vi "DetSim.vi"() -> ()   [LabVIEW 2011]
panel:
  out "Counting?":bool
  out "Count Value":dbl
  in  "stop program":bool
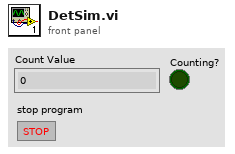
[diagram p1: front panel]
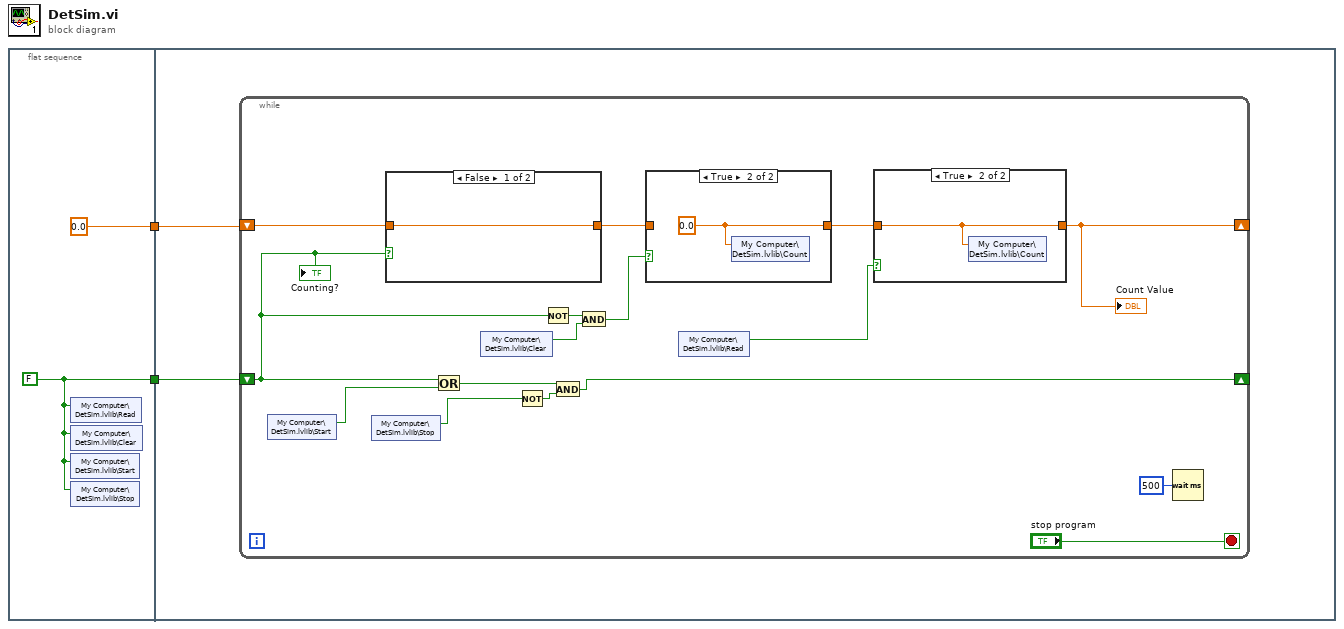
[diagram p0: block diagram]
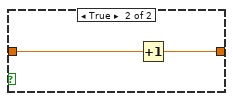
[diagram p4: hidden frame]
diagram:
  n1 = flat-sequence {
    tunnel: [0.0] -> w2
    tunnel: [w3] -> w1
    tunnel: w2 -> [w6]
    tunnel: w1 -> [w5]
    frame #0 {
      w3 = FALSE
      n2 = shared-variable "My Computer\\DetSim.lvlib\\Read"(w3) -> ()  [unwired: 1 in, 1 out]
      n3 = shared-variable "My Computer\\DetSim.lvlib\\Clear"(w3) -> ()  [unwired: 1 in, 1 out]
      n4 = shared-variable "My Computer\\DetSim.lvlib\\Start"(w3) -> ()  [unwired: 1 in, 1 out]
      n5 = shared-variable "My Computer\\DetSim.lvlib\\Stop"(w3) -> ()  [unwired: 1 in, 1 out]
    }
    frame #1 {
      n6 = while {
        shift-right: [w12] -> _
        shift-left: w6 -> [w20]
        shift-right: [w18] -> _
        shift-left: w5 -> [w14]
        stop <- "stop program" stop-if-true
        n7 = shared-variable "My Computer\\DetSim.lvlib\\Start"() -> (w10:bool)  [unwired: 1 in, 1 out]
        n8 = shared-variable "My Computer\\DetSim.lvlib\\Stop"() -> (w9:bool)  [unwired: 1 in, 1 out]
        n9 = case shown="False" w14 {
          tunnel: w20 -> [w27 w29]
          tunnel: [w27 w28] -> w16
          frame False {
          }
          frame True {
            n10 = Increment(x=w29) -> (x+1=w28:dbl)
          }
        }
        n11 = Or(x=w14, y=w10) -> (x .or. y?=w19:bool)
        n12 = shared-variable "My Computer\\DetSim.lvlib\\Clear"() -> (w8:bool)  [unwired: 1 in, 1 out]
        n13 = Not(x=w9) -> (.not. x?=w17:bool)
        n14 = Not(x=w14) -> (.not. x?=w15:bool)
        n15 = And(x=w19, y=w17) -> (x .and. y?=w18:bool)
        n16 = And(x=w15, y=w8) -> (x .and. y?=w13:bool)
        n17 = case shown="True" w13 {
          tunnel: w16 -> [w25 _]
          tunnel: [w25 w26] -> w11
          frame False {
          }
          frame True {
            w26 = 0.0
            n18 = shared-variable "My Computer\\DetSim.lvlib\\Count"(w26) -> ()  [unwired: 1 in, 1 out]
          }
        }
        n19 = shared-variable "My Computer\\DetSim.lvlib\\Read"() -> (w7:bool)  [unwired: 1 in, 1 out]
        n20 = case shown="True" w7 {
          tunnel: [w23 w24] -> w12
          tunnel: w11 -> [w23 w24]
          frame False {
          }
          frame True {
            n21 = shared-variable "My Computer\\DetSim.lvlib\\Count"(w24) -> ()  [unwired: 1 in, 1 out]
          }
        }
        "Count Value" <- w12
        n22 = Wait (ms)(milliseconds to wait=u32 500) -> ()  [unwired: 1 out]
        "Counting?" <- w14
      }
    }
  }
